vi "Close.vi"(8 "error in (no error)":errorcluster) -> (0 "error out":errorcluster)   [LabVIEW 2018, in "Covers-o-meter.lvlib"]
doc: "Enqueues named action and/or data."
uses:
  Covers-o-meter.lvlib
  Private/ctl/State--enum.ctl
  Private/ctl/Message--enum.ctl
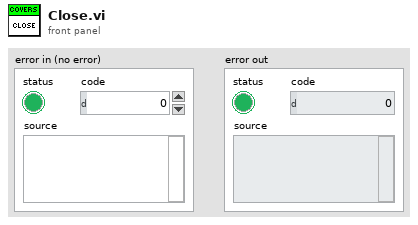
[diagram p1: front panel]
types:
  T1 = typedef "Covers-o-meter.lvlib/Message--enum.ctl" = cluster{"State":T2, "Data":variant}
  T2 = typedef "Covers-o-meter.lvlib/State--enum.ctl" = enum16{"Init", "Init: Read req tags", "Init Data: All Projects", "Init: Which Project?", "Update Requirements tags", "Get all project strings", "Search proj for tags", "Subroutine", "Update Project", "Start Button Pressed", "Start timer", "Error", "Close", "UI - Refresh Timer ", "UI - refresh graph", "UI - Refresh Tree"}
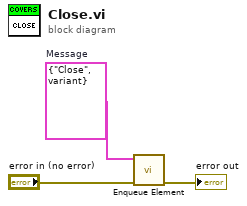
[diagram p0: block diagram]
diagram:
  w1 = T1 {"State"=enum."Close", "Data"=variant}  # Message
  n1 = call "Enqueue Element.vi"("error in"="error in (no error)", 11:w1) -> ("error out"=→"error out":errorcluster)  [unwired: 9 in]
